vi "Forward_Pass_demo.vi"() -> ()   [LabVIEW 2014]
uses:
  <vilib>/Analysis/Matrix/Datatypes/RealMatrix.ctl
  <vilib>/Analysis/baseanly.llb/Real A x B.vi
  <vilib>/Analysis/Matrix/Numeric/Add/Add - RM,RM.vi
  <vilib>/Analysis/NI_AALBase.lvlib
  <vilib>/Analysis/Matrix/NI_Matrix.lvlib
panel:
  out "output cluster":T2
  in  "by":T1
  out "Why * h":T1
  in  "Why":T1
  out "h":T1
  out "Wxh * x":T1
  in  "x":T1
  in  "Wxh":T1
  out "y":T1
  out "softmax":T1
  out "sum(e^y)":dbl
  out "e^y":T1
  in  "bh":T1
  out "Whh * h":T1
  in  "h":T1
  in  "Whh":T1
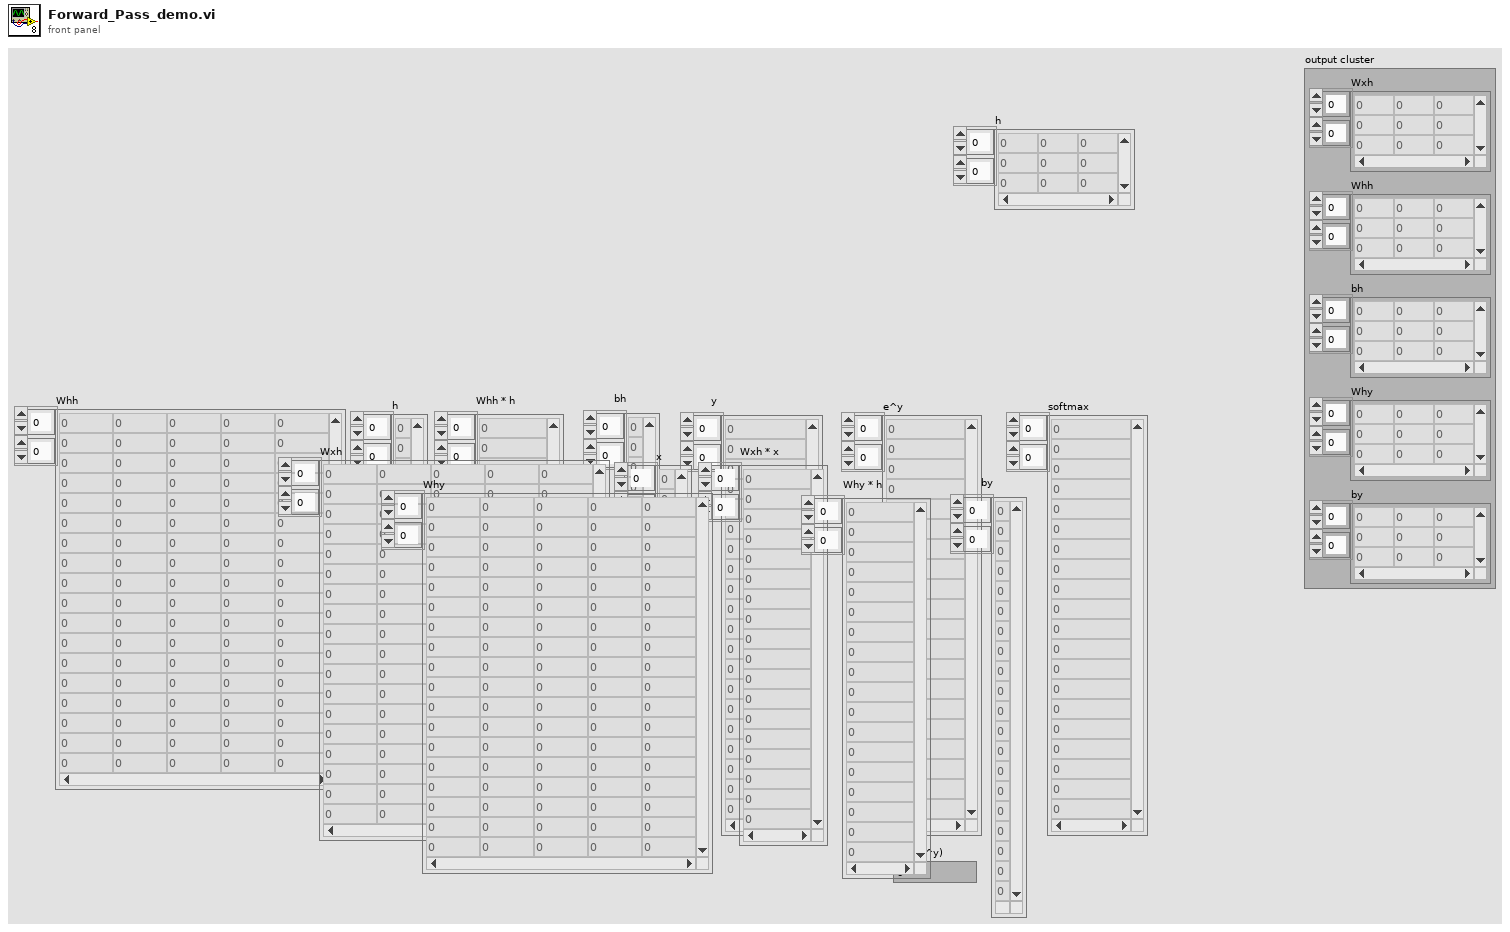
[diagram p1: front panel]
types:
  T1 = typedef "NI_Matrix.lvlib/RealMatrix.ctl" = dbl[][]
  T2 = cluster{"Wxh":T1, "Whh":T1, "bh":T1, "Why":T1, "by":T1}
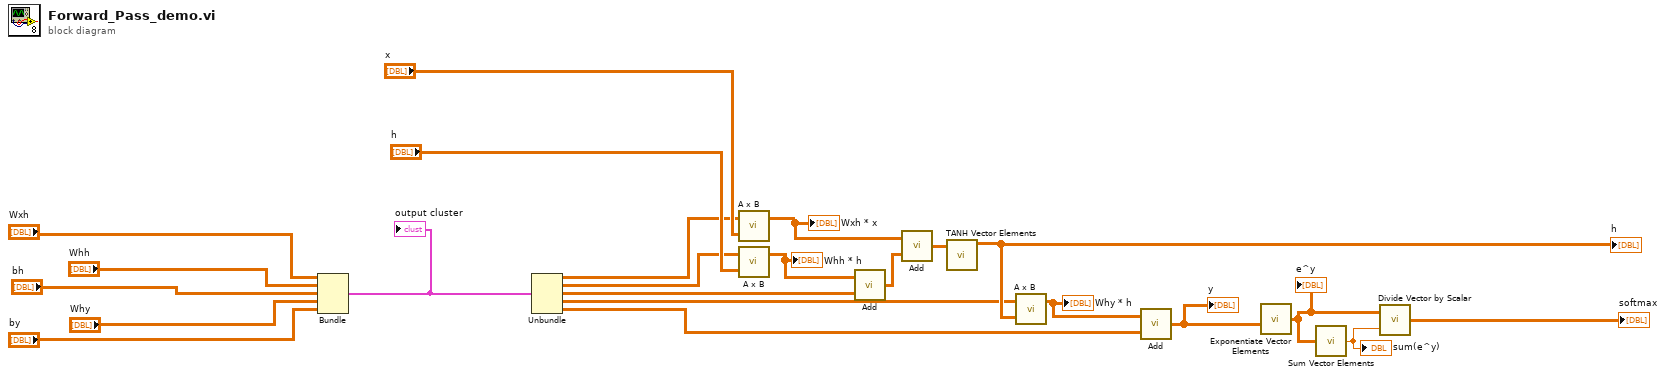
[diagram p0: block diagram]
diagram:
  n1 = Bundle("Wxh"="Wxh", "Whh"="Whh", "bh"="bh", "Why"="Why", "by"="by") -> (w6:T2)  [unwired: 1 in]
  "output cluster" <- w6
  n2 = Unbundle(w6) -> ("Wxh"=w5:T1, "Whh"=w4:T1, "bh"=w1:T1, "Why"=w2:T1, "by"=w3:T1)
  n3 = call-poly <vilib>:"A x B.vi"("B"="x", "A"=w5) -> ("A x B"=w19:T1)  [unwired: 1 out]
  "Wxh * x" <- w19
  n4 = call-poly <vilib>:"A x B.vi"("B"="h", "A"=w4) -> ("A x B"=w23:T1)  [unwired: 1 out]
  "Whh * h" <- w23
  n5 = call-poly <vilib>:"Add.vi"("Real Matrix B"=w1, "Real Matrix A"=w23) -> ("A + B"=w18:T1)
  n6 = call-poly <vilib>:"Add.vi"("Real Matrix B"=w18, "Real Matrix A"=w19) -> ("A + B"=w16:T1)
  n7 = call "TANH Vector Elements.vi"("Vector (in)"=w16) -> ("Vector (out)"=w15:T1)  [unwired: 10 in]
  "h" <- w15
  n8 = call-poly <vilib>:"A x B.vi"("B"=w15, "A"=w2) -> ("A x B"=w17:T1)  [unwired: 1 out]
  "Why * h" <- w17
  n9 = call-poly <vilib>:"Add.vi"("Real Matrix B"=w3, "Real Matrix A"=w17) -> ("A + B"=w14:T1)
  "y" <- w14
  n10 = call "Exponentiate Vector Elements.vi"("A x B"=w14) -> ("Real Matrix (Column Vector)"=w20:T1)
  "e^y" <- w20
  n11 = call "Sum Vector Elements.vi"("A x B"=w20) -> ("Numeric"=w21:dbl)
  "sum(e^y)" <- w21
  n12 = call "Divide Vector by Scalar.vi"("x"=w21, "Vector (in)"=w20) -> ("Real Matrix (Column Vector)"=→"softmax":T1)
